vi "initIRQConfig.vi"(8 "error in (no error)":errorcluster, 11 "IRQConfig in":refnum<class "IRQConfig.lvclass">) -> (0 "error out":errorcluster, 3 "IRQConfig out":refnum<class "IRQConfig.lvclass">)   [LabVIEW 2013, in "ComponentData.lvlib" / "IRQConfig.lvclass"]
uses:
  <userlib>/Common/Component/common_application/RT/ComponentData/ConfigurationHandler/IRQConfig/IRQConfig.lvclass
  <userlib>/Common/Component/common_application/MyComputer/ComponentConfiguration/ComponentConfigurationTypedefs/irqConfig.ctl
  <userlib>/Common/Component/common_application/RT/ComponentData/ConfigurationHandler/IRQConfig/IRQConfig.lvclass/IRQConfig.ctl
  <vilib>/Utility/xml.llb/Read From XML File(string).vi
  <userlib>/Common/Component/common_application/MyComputer/ComponentConfiguration.lvlib
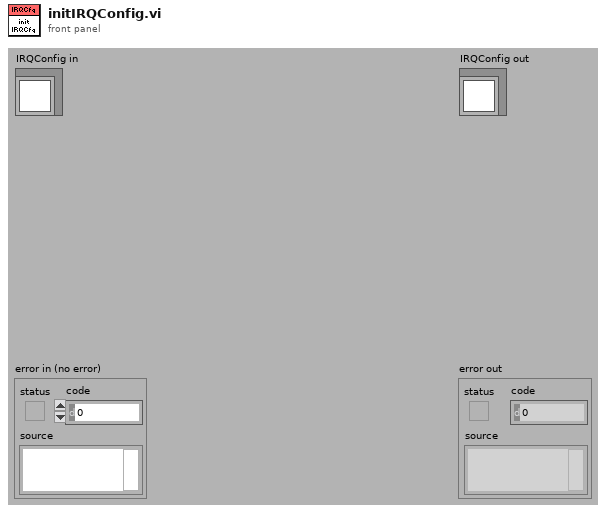
[diagram p1: front panel]
types:
  T1 = typedef "ComponentConfiguration.lvlib/irqConfig.ctl" = cluster{"irqNumber":i32, "irqTimeout_ms":i32}
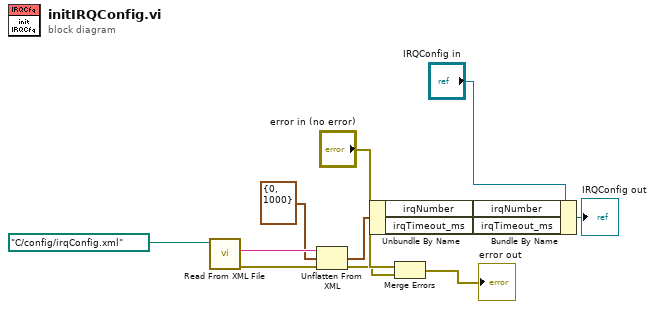
[diagram p0: block diagram]
diagram:
  n1 = call-poly <vilib>:"Read From XML File.vi"("XML File Path"=path "C:/config/irqConfig.xml" ("configuration file path")) -> ("error out"=w3:errorcluster, "XML Elements"=w9:string)  [unwired: 8 in, 1 out]
  n2 = Unflatten From XML(xml string=w9, type=T1 {"irqNumber"=0, "irqTimeout_ms"=1000} ("irqConfig"), error in (no error)=w3) -> (value=w7:T1, error out=w2:errorcluster)
  n3 = Unbundle By Name(w7) -> ("irqNumber"=w6:i32, "irqTimeout_ms"=w5:i32)
  n4 = Merge Errors("error in (no error)", w2) -> (→"error out":errorcluster)
  n5 = Bundle By Name(cluster="IRQConfig in", "irqNumber"=w6, "irqTimeout_ms"=w5) -> (→"IRQConfig out":refnum<class "IRQConfig.lvclass">)
